vi "instance count allowed.vi"(8 "error in":errorcluster, 11 "Tag Bus Web Interface configuration in":refnum<class "Tag Bus Web Interface configuration.lvclass">) -> (0 "error out":errorcluster, 2 "instances allowed":i32, 3 "Tag Bus Web Interface configuration out":refnum<class "Tag Bus Web Interface configuration.lvclass">)   [LabVIEW 2013, in "Tag Bus Web Interface configuration.lvclass"]
uses:
  Tag Bus Web Interface configuration.lvclass
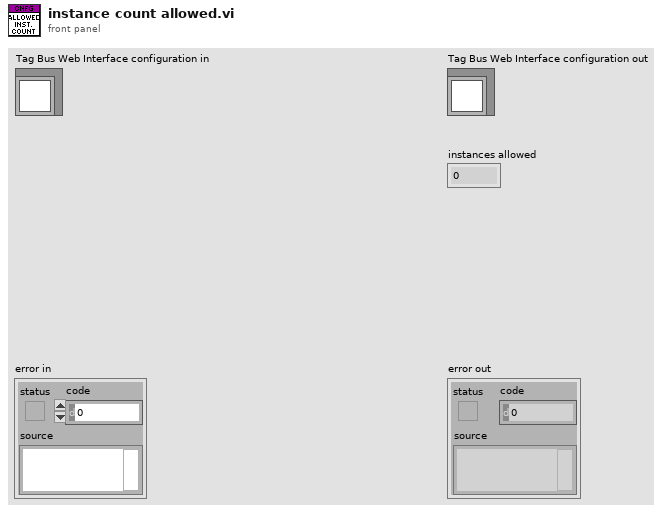
[diagram p1: front panel]
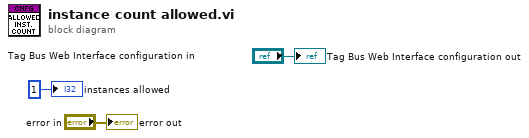
[diagram p0: block diagram]
diagram:
  "error out" <- "error in"
  "Tag Bus Web Interface configuration out" <- "Tag Bus Web Interface configuration in"
  "instances allowed" <- 1 ("instances allowed")
